vi "Weekly Superlatives.vi"(11 "Last Week's Performance vs Historical Averages":T2(array[cluster])) -> (0 "Cash Hands Played %":T1, 1 "Total Tourn Hands Won":T1, 2 "Total Tourn Hands Dealt":T1, 3 "Tourn Hands Won %":T1, 4 "Cash Hands Won %":T1, 5 "Tourn Hands Played %":T1)   [LabVIEW 2020]
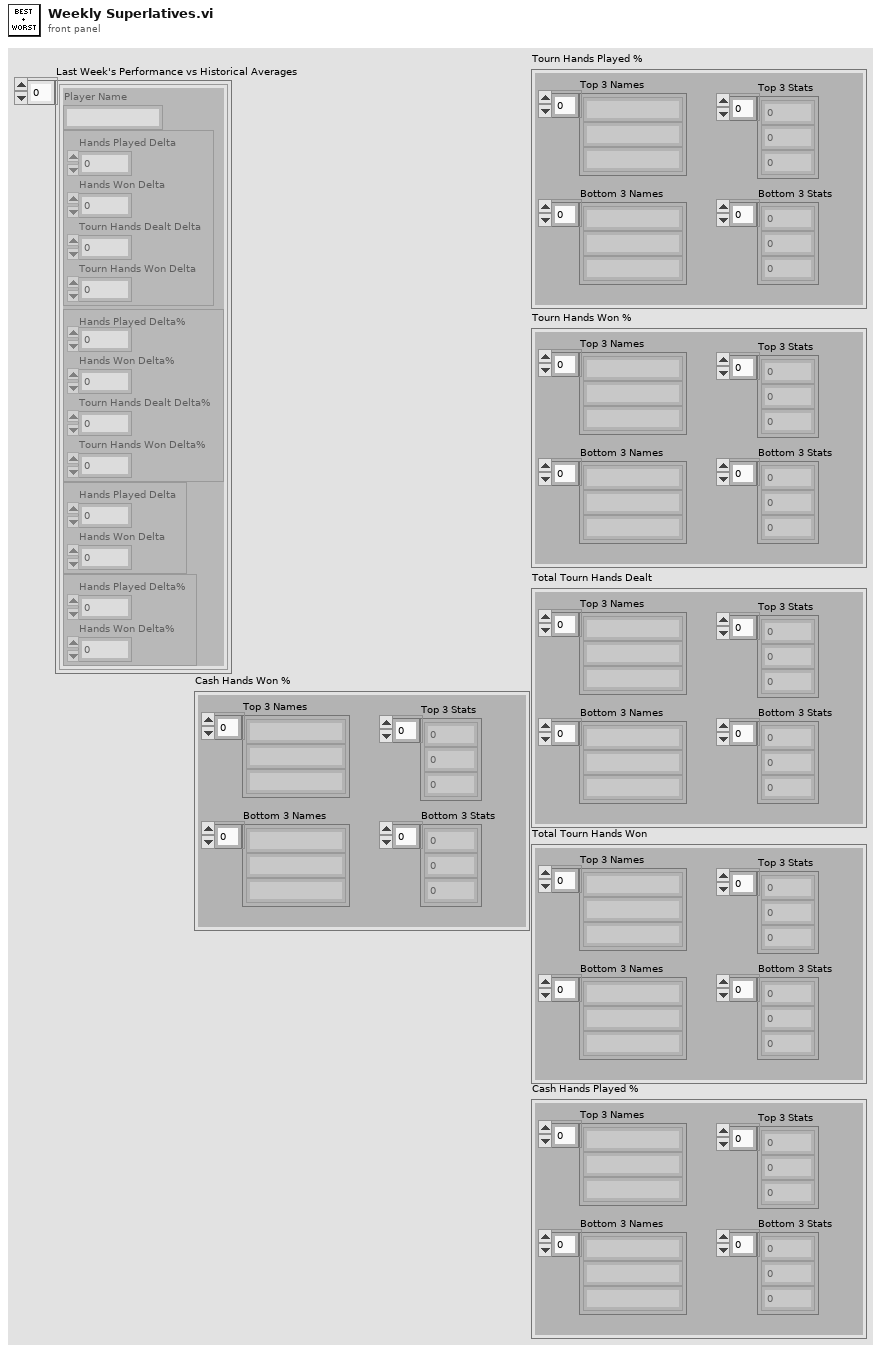
[diagram p1: front panel]
types:
  T1 = cluster{"Top 3 Names":string[], "Top 3 Stats":dbl[], "Bottom 3 Names":string[], "Bottom 3 Stats":dbl[]}
  T2 = cluster{"Player Name":string, cluster{"Hands Played Delta":dbl, "Hands Won Delta":dbl, "Tourn Hands Dealt Delta":dbl, "Tourn Hands Won Delta":dbl}, cluster{"Hands Played Delta%":dbl, "Hands Won Delta%":dbl, "Tourn Hands Dealt Delta%":dbl, "Tourn Hands Won Delta%":dbl}, cluster{"Hands Played Delta":dbl, "Hands Won Delta":dbl}, cluster{"Hands Played Delta%":dbl, "Hands Won Delta%":dbl}}[]
  T3 = cluster{"Hands Played Delta%":dbl, "Hands Won Delta%":dbl, "Tourn Hands Dealt Delta%":dbl, "Tourn Hands Won Delta%":dbl}
  T4 = cluster{"Hands Played Delta%":dbl, "Hands Won Delta%":dbl}
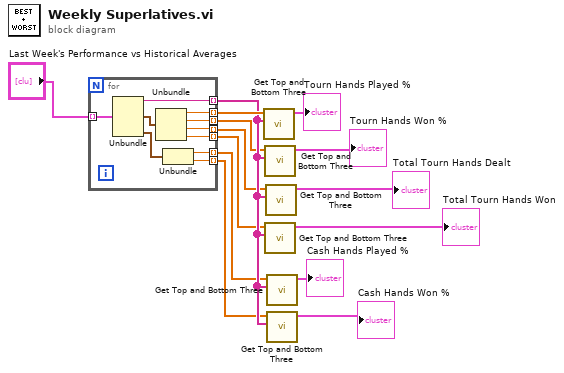
[diagram p0: block diagram]
diagram:
  n1 = for {
    tunnel: "Last Week's Performance vs Historical Averages" -> [w24] mode=indexing
    tunnel: [w23] -> w12 mode=indexing
    tunnel: [w21] -> w13 mode=indexing
    tunnel: [w20] -> w11 mode=indexing
    tunnel: [w19] -> w10 mode=indexing
    tunnel: [w18] -> w9 mode=indexing
    tunnel: [w16] -> w8 mode=indexing
    tunnel: [w15] -> w7 mode=indexing
    n2 = Unbundle(w24) -> ("Player Name"=w23:string, w22:T3, w17:T4)  [unwired: 2 out]
    n3 = Unbundle(w22) -> ("Hands Played Delta%"=w21:dbl, "Hands Won Delta%"=w20:dbl, "Tourn Hands Dealt Delta%"=w19:dbl, "Tourn Hands Won Delta%"=w18:dbl)
    n4 = Unbundle(w17) -> ("Hands Played Delta%"=w16:dbl, "Hands Won Delta%"=w15:dbl)
  }
  n5 = call "Get Top and Bottom Three.vi"("Name Array"=w12, "Stat Array"=w13) -> ("Top and Bottom 3"=→"Tourn Hands Played %":T1)  [unwired: 9 in]
  n6 = call "Get Top and Bottom Three.vi"("Name Array"=w12, "Stat Array"=w11) -> ("Top and Bottom 3"=→"Tourn Hands Won %":T1)  [unwired: 9 in]
  n7 = call "Get Top and Bottom Three.vi"("Name Array"=w12, "Stat Array"=w9) -> ("Top and Bottom 3"=→"Total Tourn Hands Won":T1)  [unwired: 9 in]
  n8 = call "Get Top and Bottom Three.vi"("Name Array"=w12, "Stat Array"=w10) -> ("Top and Bottom 3"=→"Total Tourn Hands Dealt":T1)  [unwired: 9 in]
  n9 = call "Get Top and Bottom Three.vi"("Name Array"=w12, "Stat Array"=w8) -> ("Top and Bottom 3"=→"Cash Hands Played %":T1)  [unwired: 9 in]
  n10 = call "Get Top and Bottom Three.vi"("Name Array"=w12, "Stat Array"=w7) -> ("Top and Bottom 3"=→"Cash Hands Won %":T1)  [unwired: 9 in]
